vi "Untitled 32.vi"() -> ()   [LabVIEW 2015]
uses:
  Program Files (x86)/National Instruments/LabVIEW 2015/examples/robotics/Steering/3D Omni Robot/Robot Position.ctl
  <vilib>/robotics/Steering/Wheel/Wheel Parameters.ctl
  <vilib>/robotics/Steering/Wheel/Rotation Direction.ctl
  <vilib>/Simulation/Scripting/Companion Diagram/SimConfigNode/SimParams.ctl
  <vilib>/Simulation/Scripting/Companion Diagram/SimConfigNode/_simSolvers.ctl
  <vilib>/Simulation/Implementation/Shared/SIMSCR Execution Mode.ctl
  <vilib>/Platform/TimedLoop/XDataNode/timing_clust.ctl
  <vilib>/Platform/TimedLoop/XDataNode/nitl_modes.ctl
  <vilib>/Platform/TimedLoop/XDataNode/wakeup.ctl
  <vilib>/Simulation/Param Hierarchy/Typedefs/SIMPH Param Control Actions.ctl
  <vilib>/Simulation/Implementation/Shared/NILVSim_ParamChanged.vi
  <vilib>/Simulation/Implementation/Shared/NILVSim_FinishedLate.vi
  <vilib>/Simulation/Implementation/Shared/NILVSIM_BeginStep.vi
  <vilib>/Simulation/Utility/Implementation/SIM Halt.vi
  <vilib>/Simulation/Implementation/Shared/NILVSim_Manager.vi
  <vilib>/Utility/error.llb/Clear Errors.vi
  <vilib>/Simulation/Implementation/Shared/NILVSim_FinalizeModel.vi
  <vilib>/Analysis/coordinate.llb/2D Cartesian Coordinate Rotation.vi
  <vilib>/Analysis/coordinate.llb/2D Cartesian Coordinate Rotation (Scalar).vi
  <vilib>/robotics/Steering/Omnidirectional Wheel/Create Omnidirectional Wheel.vi
  <vilib>/robotics/Steering/Steering Frame/Create User Defined Steering Frame.vi
  <vilib>/Simulation/Implementation/Shared/SIM Unbundle Sim Info.vi
  <vilib>/Simulation/Implementation/Shared/SIMSH Read Queue.vi
  <vilib>/Simulation/Implementation/Shared/NILVSim_Initialize.vi
  <vilib>/Simulation/Utility/Implementation/NILVSim Get Time and IsAcceptedStep.vi
  <vilib>/Simulation/Implementation/Shared/NILVSim_GetModelError.vi
  <vilib>/Simulation/Implementation/Shared/SIM Bundle Sim Info.vi
  <vilib>/robotics/Steering/Steering Frame/Apply Steering Frame Velocity to Motors.vi
  <vilib>/robotics/Steering/Steering Frame/Get Steering Frame Velocity from Motors.vi
  <vilib>/Simulation/Scripting/Companion Diagram/SimConfigNode/SimDog.xnode
  Program Files (x86)/National Instruments/LabVIEW 2015/examples/robotics/Steering/3D Omni Robot/Omni Robot Model.vi
  <vilib>/Platform/TimedLoop/XDataNode/XDataNode.xnode
  <vilib>/Simulation/Implementation/XNodeFramework/SimXNode/SimX.xnode
  <vilib>/robotics/Steering/Steering Frame/NI_Robotics_Steering Frame.lvclass
  <vilib>/robotics/Steering/Wheel/NI_Robotics_Wheel.lvclass
  <vilib>/robotics/Steering/Omnidirectional Wheel/NI_Robotics_Omnidirectional Wheel.lvclass
  <vilib>/Platform/TimedLoop/XDataNode/XDNodeRunTimeDep.lvlib
  <vilib>/Simulation/Implementation/Shared/NI_SIM_Implementation.lvlib
panel:
  out "complete":bool
  in  "X Velocity (m/s)":dbl(slide) min=-1.0 max=1.0 scale=-1.0..1.0
  in  "Y Velocity (m/s)":dbl(slide) min=-1.0 max=1.0 scale=-1.0..1.0
  in  "Angular Velocity (rad/s)":dbl(slide) min=-1.0 max=1.0 scale=1.0..-1.0
  out "X Velocity Feedback":dbl(slide) scale=-1.0..1.0
  out "Y Velocity Feedback":dbl(slide) scale=-1.0..1.0
  out "Angular Velocity Feedback":dbl(slide) scale=1.0..-1.0
  in  "stop":bool
  in  "Velocity":T1(ring)
  out "robot position":T2 {"ccw wheel angles" format="%#.3f"; "global theta" format="%#.3f"; "global y" format="%#.3f"; "global x" format="%#.3f"}
  in  "reset":bool
  in  "motor setpoints":dbl[](array[numeric])=[0.0, 0.0, 0.0] format="%#.3f"
  out "motor states":dbl[](array[numeric]) format="%#.3f"
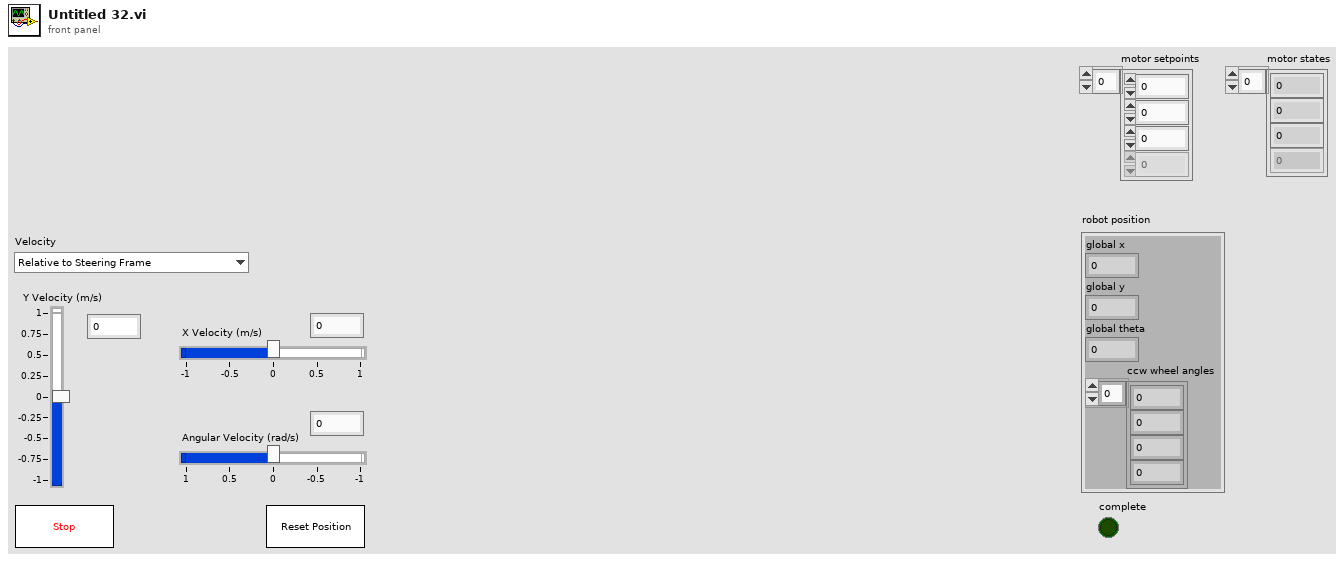
[diagram p1: front panel]
types:
  T1 = enum16{"Relative to Steering Frame", "Relative to Global Frame"}
  T2 = typedef "Robot Position.ctl" = cluster{"global x":dbl, "global y":dbl, "global theta":dbl, "ccw wheel angles":dbl[]}
  T3 = typedef "NI_Robotics_Wheel.lvclass/Rotation Direction.ctl" = u16
  T4 = typedef "NI_Robotics_Wheel.lvclass/Wheel Parameters.ctl" = cluster{"wheel radius":dbl, "gear ratio":dbl, "forward rotation direction":T3}
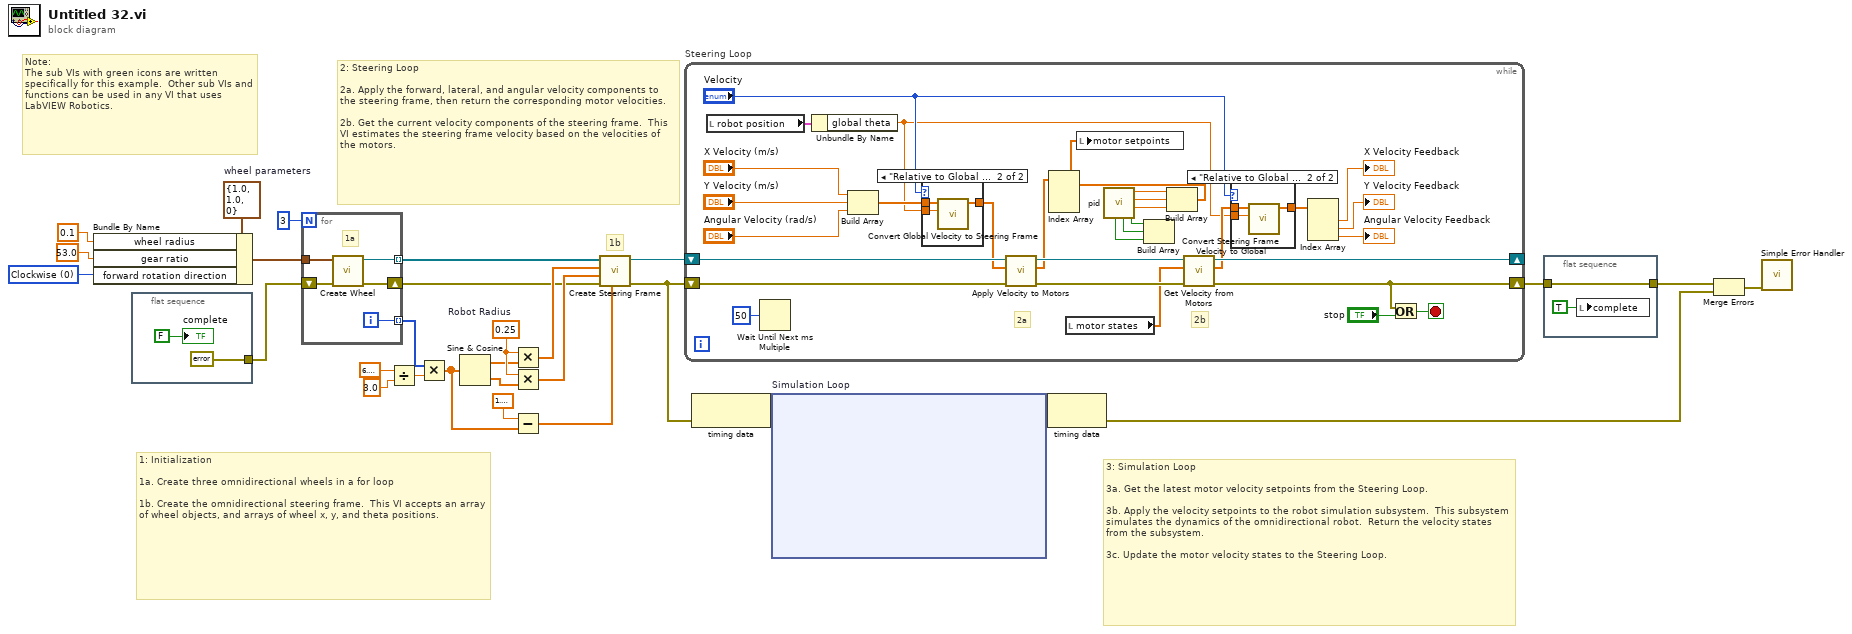
[diagram p0: block diagram]
diagram:
  w8 = T3 0 items=["Clockwise", "Counterclockwise"] ("forward rotation direction")
  w13 = 0.25  # Robot Radius
  w26 = T4 {"wheel radius"=1.0, "gear ratio"=1.0, "forward rotation direction"=0}  # wheel parameters
  # "3: Simulation Loop\n\n3a. Get the latest motor velocity setpoints from the Steering Loop.\n\n3b. Apply the velocity setpoints to the robot simulation subsystem.  This subsystem simulates the dynamics of the omnidirectional robot.  Return the velocity states from the subsystem.\n\n3c. Update the motor velocity states to the Steering Loop."
  # "Note:\nThe sub VIs with green icons are written specifically for this example.  Other sub VIs and functions can be used in any VI that uses LabVIEW Robotics."
  # "2: Steering Loop\n\n2a. Apply the forward, lateral, and angular velocity components to the steering frame, then return the corresponding motor velocities.\n\n2b. Get the current velocity components of the steering frame.  This VI estimates the steering frame velocity based on the velocities of the motors."
  # "1b"
  # "1: Initialization\n\n1a. Create three omnidirectional wheels in a for loop\n\n1b. Create the omnidirectional steering frame.  This VI accepts an array of wheel objects, and arrays of wheel x, y, and theta positions."
  n1 = Bundle By Name(cluster=w26, "wheel radius"=0.1, "gear ratio"=53.0, "forward rotation direction"=w8) -> (w23:T4)
  n2 = flat-sequence {
    tunnel: [errorcluster {"status"=FALSE, "code"=0, "source"=""} ("error out")] -> w21
    frame #0 {
      "complete" <- FALSE ("complete")
    }
  }
  n3 = for {
    N: 3 -> [_]
    shift-right: [w35] -> w5
    shift-left: w21 -> [w36]
    tunnel: [w34] -> w18 mode=indexing
    tunnel: w23 -> [w33]
    tunnel: [w32] -> w14 mode=indexing
    i -> [w32]
    # "1a"
    n4 = call-poly <vilib>:"Create Wheel.vi"("error in (no error)"=w36, "wheel parameters"=w33) -> ("error out"=w35:errorcluster, "omni wheel out"=w34:refnum<class "NI_Robotics_Omnidirectional Wheel.lvclass">)  [unwired: 8 in]
  }
  n5 = Divide(x=6.283185307179586, y=3.0) -> (x/y=w15:dbl)
  n6 = Multiply(x=w14, y=w15) -> (x*y=w3:dbl[])
  n7 = Sine & Cosine(0:w3) -> (1:w2:dbl[], 2:w1:dbl[])
  n8 = Multiply(x=w13, y=w2) -> (x*y=w12:dbl[])
  n9 = Multiply(x=w13, y=w1) -> (x*y=w11:dbl[])
  n10 = Subtract(x=1.5707963267948966, y=w3) -> (x-y=w9:dbl[])
  n11 = call-poly <vilib>:"Create Steering Frame.vi"("wheel frame angles (rad)"=w9, "error in (no error)"=w5, "wheel y positions"=w11, "wheel x positions"=w12, "wheels"=w18) -> ("error out"=w4:errorcluster, "steering frame out"=w27:refnum<class "NI_Robotics_Steering Frame.lvclass">)  [unwired: 5 in]
  n12 = while "Steering Loop" {
    shift-right: [w54] -> _
    shift-left: w27 -> [w57]
    shift-right: [w46] -> w22
    shift-left: w4 -> [w56]
    stop <- w59 stop-if-true
    # "2b"
    # "2a"
    n13 = local read "robot position"() -> (w48:T2)
    n14 = Wait Until Next ms Multiple(millisecond multiple=u32 50) -> ()  [unwired: 1 out]
    n15 = Unbundle By Name(w48) -> ("global theta"=w47:dbl)
    n16 = Build Array("X Velocity (m/s)", "Y Velocity (m/s)", "Angular Velocity (rad/s)") -> (w52:dbl[])
    n17 = case shown="\"Relative to Global Frame\"" "Velocity" {
      tunnel: w52 -> [w72 w75]
      tunnel: [w72 w74] -> w51
      tunnel: w47 -> [_ w73]
      frame "Relative to Steering Frame", Default {
      }
      frame "Relative to Global Frame" {
        n18 = call <vilib>:"Convert Global Velocity to Steering Frame.vi"("steering frame angle (rad)"=w73, "global velocity"=w75) -> ("steering frame velocity"=w74:dbl[])  [unwired: 9 in]
      }
    }
    n19 = call-poly <vilib>:"Apply Velocity to Motors.vi"("error in (no error)"=w56, "steering frame velocity"=w51, "steering frame in"=w57) -> ("error out"=w55:errorcluster, "ccw motor velocity setpoints"=w45:dbl[], "steering frame out"=w58:refnum<class "NI_Robotics_Steering Frame.lvclass">)  [unwired: 4 in, 2 out]
    n20 = Index Array(array=w45) -> ()  [unwired: 3 in, 3 out]
    n21 = local read "motor states"() -> (w38:dbl[])
    n22 = call "pid.vi"() -> ("Direct M3"=w41:bool, "Pwm M3"=w42:dbl, "Pwm M2"=w43:dbl, "Pwm M1"=w44:dbl, "Direct M2"=w40:bool, "Direct M1"=w39:bool)  [unwired: 3 in, 3 out]
    n23 = Build Array(w41, w40, w39) -> ()  [unwired: 1 out]
    n24 = Build Array(w44, w43, w42) -> (w37:dbl[])
    n25 = local write "motor setpoints"(w37) -> ()
    n26 = call-poly <vilib>:"Get Velocity from Motors.vi"("error in (no error)"=w55, "ccw motor velocity states"=w38, "steering frame in"=w58) -> ("error out"=w46:errorcluster, "estimated steering frame velocity"=w50:dbl[], "steering frame out"=w54:refnum<class "NI_Robotics_Steering Frame.lvclass">)  [unwired: 6 in]
    n27 = case shown="\"Relative to Global Frame\"" "Velocity" {
      tunnel: w50 -> [w68 w71]
      tunnel: [w68 w70] -> w49
      tunnel: w47 -> [_ w69]
      frame "Relative to Steering Frame", Default {
      }
      frame "Relative to Global Frame" {
        n28 = call <vilib>:"Convert Steering Frame Velocity to Global.vi"("steering frame angle (rad)"=w69, "steering frame velocity"=w71) -> ("global velocity"=w70:dbl[])  [unwired: 9 in]
      }
    }
    n29 = Index Array(array=w49) -> (element #1=→"X Velocity Feedback":dbl, element #2=→"Y Velocity Feedback":dbl, element #3=→"Angular Velocity Feedback":dbl)  [unwired: 3 in]
    n30 = Or(x=w46, y="stop") -> (x .or. y?=w59:bool)
  }
  n31 = node-c288(w4) -> (w29:variant)
  n32 = node-c254 "Simulation Loop"(w29) -> (w28:variant)
  n33 = node-c288(w28) -> (w6:errorcluster)
  n34 = flat-sequence {
    tunnel: w22 -> [w76]
    tunnel: [w76] -> w20
    frame #0 {
      n35 = local write "complete"(TRUE ("complete")) -> ()
    }
  }
  n36 = Merge Errors(w20, w6) -> (w19:errorcluster)
  n37 = call <vilib>:"Simple Error Handler.vi"("error in (no error)"=w19) -> ()  [unwired: 4 in, 5 out]
